vi "FTW-JSON-Array-Deserialize.vi"(5 "Array of JSON Objects":string, 11 "error in":errorcluster) -> (6 "JSON Elements":string[](array[string]), 8 "Valid Structure":bool, 15 "error out":errorcluster)   [LabVIEW 2012]
uses:
  Regex/FTW-Regex.vi
  FTW-JSON-RegexHeader.vi
  Error/FTW-ERR-ThrowError.vi
panel:
  # "Inputs"
  # "Outputs"
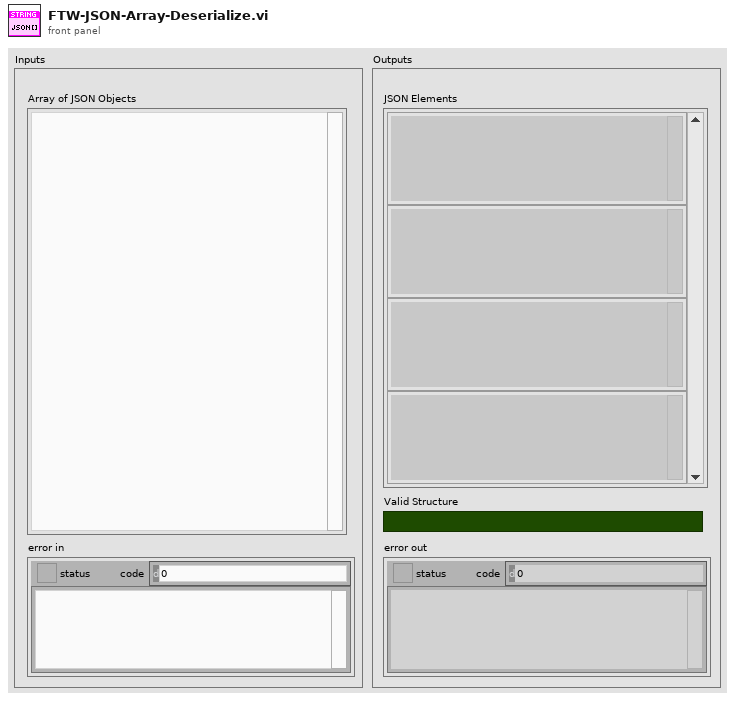
[diagram p1: front panel]
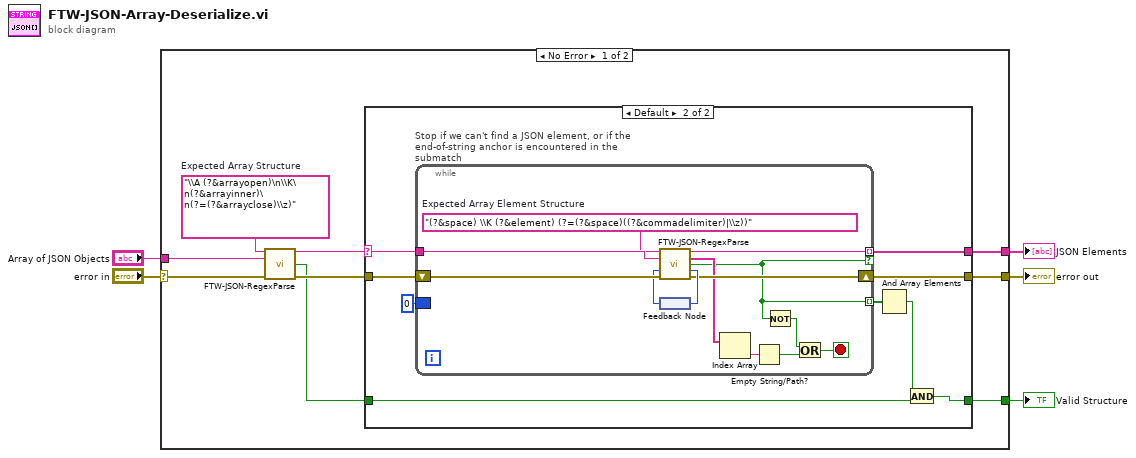
[diagram p0: block diagram]
diagram:
  n1 = case shown="No Error" "error in" {
    selector: "error in" -> [w10 w39]
    tunnel: [w13 w39] -> w5
    tunnel: [w12 _] -> w4
    tunnel: [w9 _] -> w3
    tunnel: "Array of JSON Objects" -> [w11 _]
    frame No Error {
      w7 = "\\A (?&arrayopen)\n\\K\n(?&arrayinner)\n(?=(?&arrayclose)\\z)"  # Expected Array Structure
      n2 = call "FTW-JSON-RegexParse.vi"("Regular Expression using JSON subroutines"=w7, "Input String"=w11, "error in"=w10) -> ("Match"=w6:string, "Found Match?"=w8:bool, "error out"=w14:errorcluster)  [unwired: 8 in, 2 out]
      n3 = case shown="Default" w6 {
        selector: w6 -> [_ w17]
        tunnel: w14 -> [w16 w25]
        tunnel: [w16 w24] -> w13
        tunnel: [_ w23] -> w12
        tunnel: [w15 w22] -> w9
        tunnel: w8 -> [w15 w21]
        frame "" {
        }
        frame Default {
          n4 = while "Stop if we can't find a JSON element, or if the\nend-of-string anchor is encountered in the submatch" {
            tunnel: w17 -> [w37]
            shift-right: [w34] -> w24
            shift-left: w25 -> [w38]
            tunnel: [w35] -> w23 mode=indexing if=w28
            border: 0 -> [_]
            tunnel: [w28] -> w19 mode=indexing
            stop <- w29 stop-if-true
            w27 = "(?&space) \\K (?&element) (?=(?&space)((?&commadelimiter)|\\z))"  # Expected Array Element Structure
            n5 = feedback #1() -> (w26:i32)
            n6 = call "FTW-JSON-RegexParse.vi"("Regular Expression using JSON subroutines"=w27, "Input String"=w37, "Starting Offset"=w26, "error in"=w38) -> ("Match"=w35:string, "Submatches"=w33:string[], "Found Match?"=w28:bool, "Offset after Match"=w36:i32, "error out"=w34:errorcluster)  [unwired: 7 in]
            n7 = feedback-in #1(w36) -> ()
            n8 = Index Array(array=w33) -> (element=w32:string)  [unwired: 1 in]
            n9 = Empty String/Path?(string/path=w32) -> (empty?=w31:bool)
            n10 = Not(x=w28) -> (.not. x?=w30:bool)
            n11 = Or(x=w30, y=w31) -> (x .or. y?=w29:bool)
          }
          n12 = And Array Elements(Boolean array=w19) -> (logical AND=w18:bool)
          n13 = And(x=w18, y=w21) -> (x .and. y?=w22:bool)
        }
      }
    }
    frame Error {
    }
  }
  "JSON Elements" <- w4
  "error out" <- w5
  "Valid Structure" <- w3
